vi "ModbusCmdIn.vi"(8 "error in (no error)":errorcluster, 10 "data":T1, 11 "Enum":T2) -> (0 "error out":errorcluster)   [LabVIEW 2019]
uses:
  Ctrl/ModbusCmd.ctl
  Subvi/RobotControlQueueIn.vi
panel:
  out "data 2":T1
  in  "variant 3":variant
  in  "Data":variant
  out "variant 2":variant
  out "variant":variant
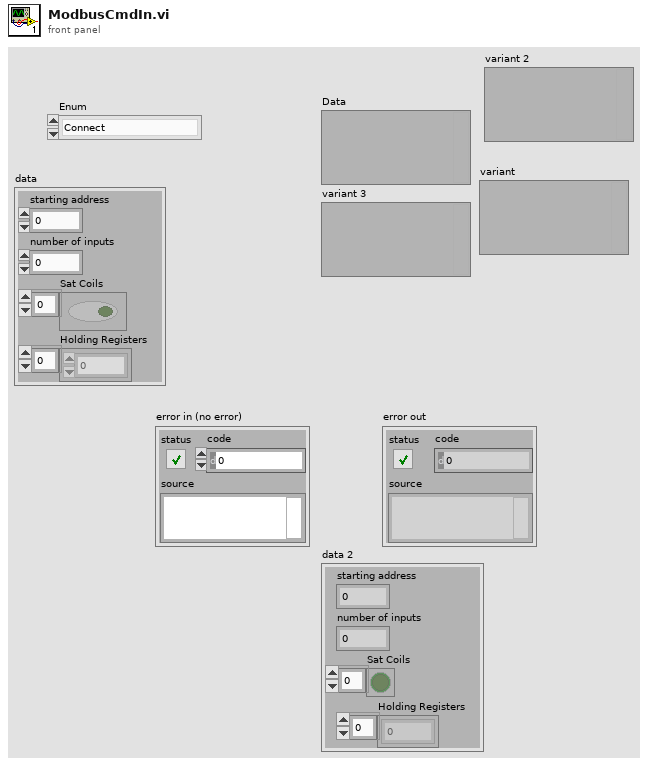
[diagram p1: front panel]
types:
  T1 = cluster{"starting address":u16, "number of inputs":u16, "Sat Coils":bool[], "Holding Registers":u16[]}
  T2 = typedef "ModbusCmd.ctl" = enum16{"Connect", "Disconnect", "Init", "Fetch Basic Objects", "Fetch Input Refisters", "Fetch Discrete Inputs", "Set Coils", "Set Holding Registers", "Write Single Holding", "Exit"}
  T3 = cluster{"starting address":u16, "number of inputs":u16, "Sat Coils":bool[]}
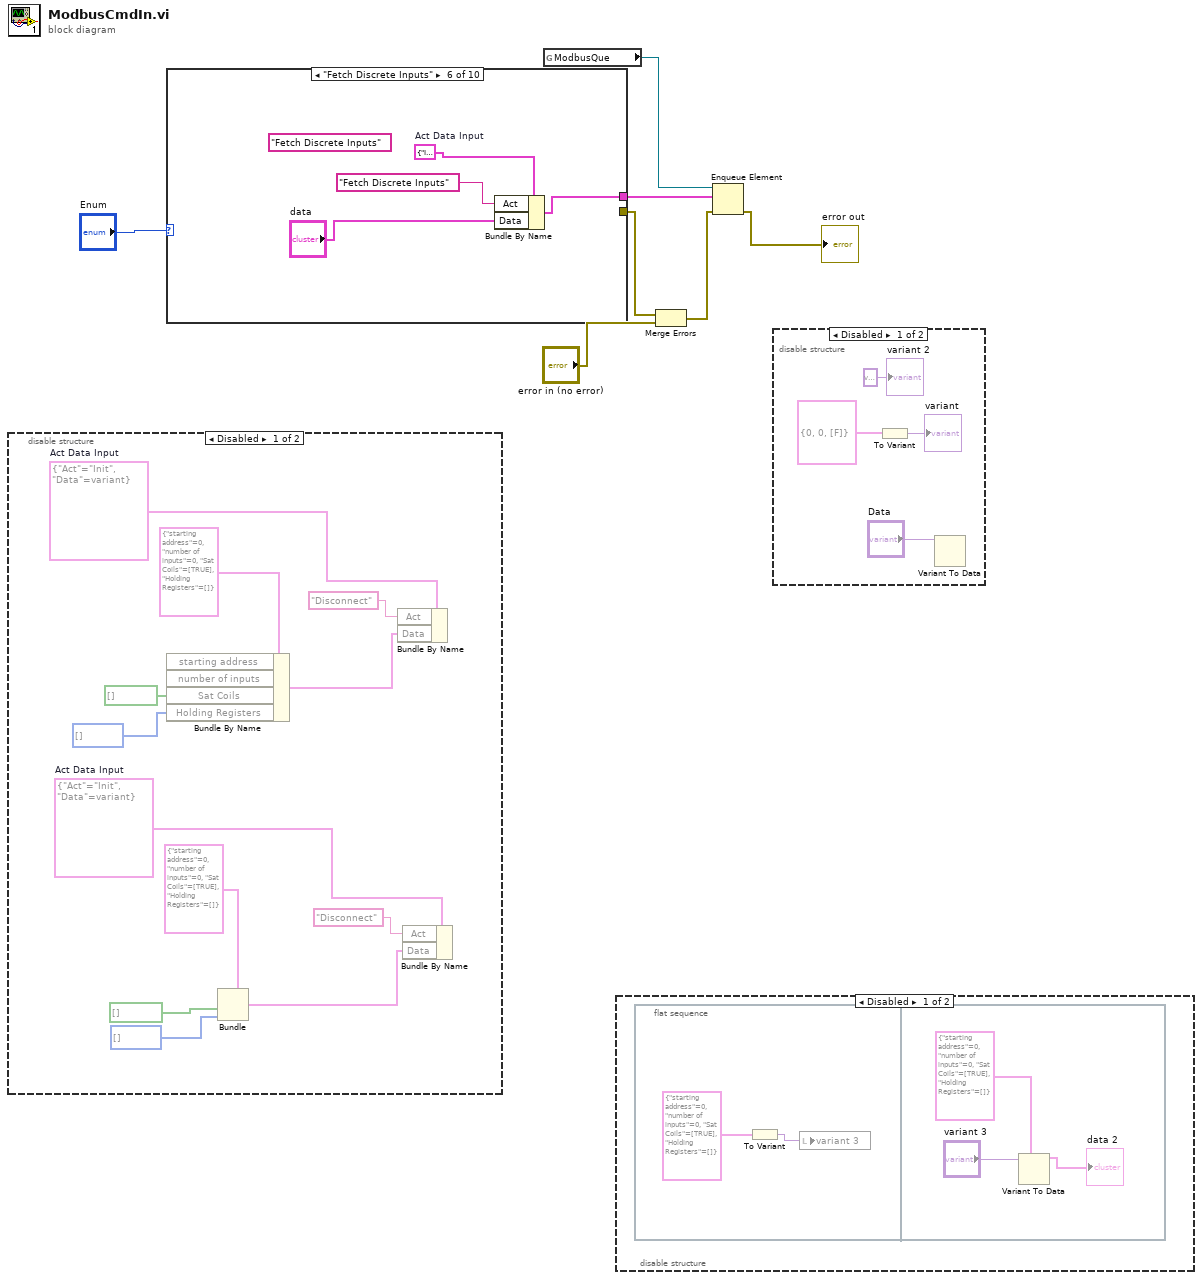
[diagram p0: block diagram]
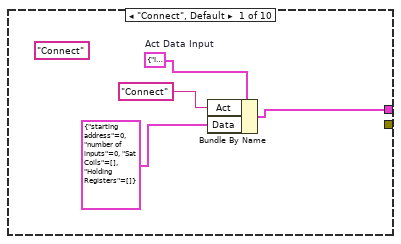
[diagram p5: hidden frame]
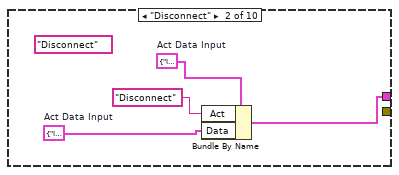
[diagram p6: hidden frame]
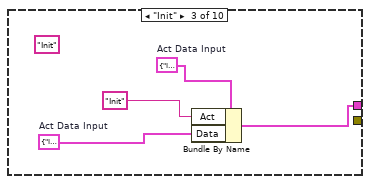
[diagram p7: hidden frame]
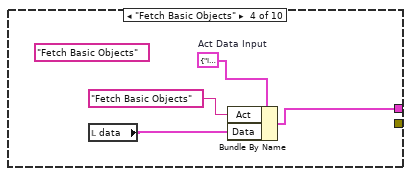
[diagram p8: hidden frame]
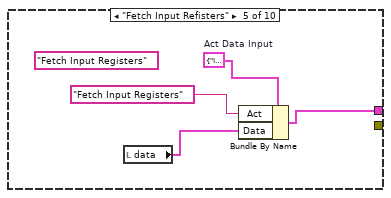
[diagram p9: hidden frame]
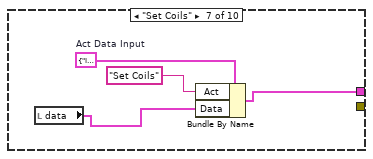
[diagram p10: hidden frame]
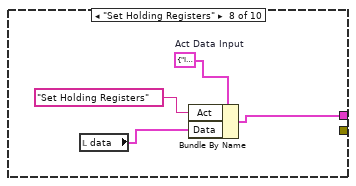
[diagram p11: hidden frame]
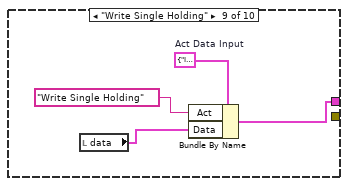
[diagram p12: hidden frame]
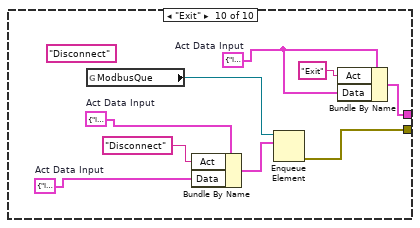
[diagram p13: hidden frame]
diagram:
  n1 = disable-structure shown="Disabled" {
    frame Disabled {
      w9 = cluster{"Act":string, "Data":variant} {"Act"="Init", "Data"=variant}  # Act Data Input
      w18 = cluster{"Act":string, "Data":variant} {"Act"="Init", "Data"=variant}  # Act Data Input
      n2 = Bundle By Name(cluster=T1 {"starting address"=0, "number of inputs"=0, "Sat Coils"=[TRUE], "Holding Registers"=[]} ("data"), "Sat Coils"=bool[] [], "Holding Registers"=u16[] []) -> (w17:T1)  [unwired: 2 in]
      n3 = Bundle(cluster=T1 {"starting address"=0, "number of inputs"=0, "Sat Coils"=[TRUE], "Holding Registers"=[]} ("data"), "Sat Coils"=bool[] [], "Holding Registers"=u16[] []) -> (w10:T1)  [unwired: 2 in]
      n4 = Bundle By Name(cluster=w18, "Act"="Disconnect", "Data"=w17) -> ()  [unwired: 1 out]
      n5 = Bundle By Name(cluster=w9, "Act"="Disconnect", "Data"=w10) -> ()  [unwired: 1 out]
    }
    frame Enabled {
    }
  }
  n6 = case shown="\"Fetch Discrete Inputs\"" "Enum" {
    tunnel: [w22 w26 w30 w34 w38 w42 w46 w50 w52 w59] -> w2
    tunnel: [_ _ _ _ _ _ _ _ _ w63] -> w4
    frame "Connect", Default {
      w21 = cluster{"Act":string, "Data":variant} {"Act"="Init", "Data"=variant}  # Act Data Input
      (unwired) "Connect" ("element")
      n7 = Bundle By Name(cluster=w21, "Act"="Connect", "Data"=T1 {"starting address"=0, "number of inputs"=0, "Sat Coils"=[], "Holding Registers"=[]} ("data")) -> (w22:cluster{"Act":string, "Data":variant})
    }
    frame "Disconnect" {
      w24 = cluster{"Act":string, "Data":variant} {"Act"="Init", "Data"=variant}  # Act Data Input
      w25 = cluster{"Act":string, "Data":variant} {"Act"="Init", "Data"=variant}  # Act Data Input
      (unwired) "Disconnect" ("element")
      n8 = Bundle By Name(cluster=w25, "Act"="Disconnect", "Data"=w24) -> (w26:cluster{"Act":string, "Data":variant})
    }
    frame "Init" {
      w28 = cluster{"Act":string, "Data":variant} {"Act"="Init", "Data"=variant}  # Act Data Input
      w29 = cluster{"Act":string, "Data":variant} {"Act"="Init", "Data"=variant}  # Act Data Input
      (unwired) "Init" ("element")
      n9 = Bundle By Name(cluster=w29, "Act"="Init", "Data"=w28) -> (w30:cluster{"Act":string, "Data":variant})
    }
    frame "Fetch Basic Objects" {
      w33 = cluster{"Act":string, "Data":variant} {"Act"="Init", "Data"=variant}  # Act Data Input
      (unwired) "Fetch Basic Objects" ("element")
      n10 = local read "data"() -> (w32:T1)
      n11 = Bundle By Name(cluster=w33, "Act"="Fetch Basic Objects", "Data"=w32) -> (w34:cluster{"Act":string, "Data":variant})
    }
    frame "Fetch Input Refisters" {
      w37 = cluster{"Act":string, "Data":variant} {"Act"="Init", "Data"=variant}  # Act Data Input
      (unwired) "Fetch Input Registers" ("element")
      n12 = local read "data"() -> (w36:T1)
      n13 = Bundle By Name(cluster=w37, "Act"="Fetch Input Registers", "Data"=w36) -> (w38:cluster{"Act":string, "Data":variant})
    }
    frame "Fetch Discrete Inputs" {
      w41 = cluster{"Act":string, "Data":variant} {"Act"="Init", "Data"=variant}  # Act Data Input
      (unwired) "Fetch Discrete Inputs" ("element")
      n14 = Bundle By Name(cluster=w41, "Act"="Fetch Discrete Inputs", "Data"="data") -> (w42:cluster{"Act":string, "Data":variant})
    }
    frame "Set Coils" {
      w44 = cluster{"Act":string, "Data":variant} {"Act"="Init", "Data"=variant}  # Act Data Input
      n15 = local read "data"() -> (w45:T1)
      n16 = Bundle By Name(cluster=w44, "Act"="Set Coils", "Data"=w45) -> (w46:cluster{"Act":string, "Data":variant})
    }
    frame "Set Holding Registers" {
      w49 = cluster{"Act":string, "Data":variant} {"Act"="Init", "Data"=variant}  # Act Data Input
      n17 = local read "data"() -> (w48:T1)
      n18 = Bundle By Name(cluster=w49, "Act"="Set Holding Registers", "Data"=w48) -> (w50:cluster{"Act":string, "Data":variant})
    }
    frame "Write Single Holding" {
      w54 = cluster{"Act":string, "Data":variant} {"Act"="Init", "Data"=variant}  # Act Data Input
      n19 = local read "data"() -> (w55:T1)
      n20 = Bundle By Name(cluster=w54, "Act"="Write Single Holding", "Data"=w55) -> (w52:cluster{"Act":string, "Data":variant})
    }
    frame "Exit" {
      w56 = cluster{"Act":string, "Data":variant} {"Act"="Init", "Data"=variant}  # Act Data Input
      w57 = cluster{"Act":string, "Data":variant} {"Act"="Init", "Data"=variant}  # Act Data Input
      w58 = cluster{"Act":string, "Data":variant} {"Act"="Init", "Data"=variant}  # Act Data Input
      (unwired) "Disconnect" ("element")
      n21 = global read "RobotControlQueueIn.vi" "ModbusQue"() -> (w64:refnum<queue>)
      n22 = Bundle By Name(cluster=w57, "Act"="Disconnect", "Data"=w58) -> (w61:cluster{"Act":string, "Data":variant})
      n23 = Enqueue Element(queue=w64, element=w61) -> (error out=w63:errorcluster)  [unwired: 2 in, 2 out]
      n24 = Bundle By Name(cluster=w56, "Act"="Exit" ("element"), "Data"=w56) -> (w59:cluster{"Act":string, "Data":variant})
    }
  }
  n25 = global read "RobotControlQueueIn.vi" "ModbusQue"() -> (w7:refnum<queue>)
  n26 = disable-structure shown="Disabled" {
    frame Disabled {
      n27 = flat-sequence {
        frame #0 {
          n28 = To Variant(anything=T1 {"starting address"=0, "number of inputs"=0, "Sat Coils"=[TRUE], "Holding Registers"=[]} ("data")) -> (Variant=w65:variant)
          n29 = local write "variant 3"(w65) -> ()
        }
        frame #1 {
          n30 = Variant To Data(type=T1 {"starting address"=0, "number of inputs"=0, "Sat Coils"=[TRUE], "Holding Registers"=[]} ("data"), Variant="variant 3") -> (data=→"data 2":T1)  [unwired: 1 in, 1 out]
        }
      }
    }
    frame Enabled {
    }
  }
  n31 = Merge Errors(w4, "error in (no error)") -> (w3:errorcluster)
  n32 = Enqueue Element(queue=w7, element=w2, error in (no error)=w3) -> (error out=→"error out":errorcluster)  [unwired: 1 in, 2 out]
  n33 = disable-structure shown="Disabled" {
    frame Disabled {
      n34 = To Variant(anything=T3 {"starting address"=0, "number of inputs"=0, "Sat Coils"=[FALSE]} ("output cluster 2")) -> (Variant=→"variant":variant)
      n35 = Variant To Data(Variant="Data") -> ()  [unwired: 2 in, 2 out]
      "variant 2" <- variant ("variant 2")
    }
    frame Enabled {
    }
  }
